vi "Write Resource.vi"(8 "error in (no error)":errorcluster, 10 "Resource":refnum<visa-resource-name>, 11 "Oscilloscope in":refnum<class "Oscilloscope.lvclass">) -> (0 "error out":errorcluster, 3 "Oscilloscope out":refnum<class "Oscilloscope.lvclass">)   [LabVIEW 2018, in "Oscilloscope.lvlib" / "Oscilloscope.lvclass"]
doc: "This acessor method writes resource ID setting."
uses:
  Oscilloscope.lvclass
  Oscilloscope.lvclass/Oscilloscope.ctl
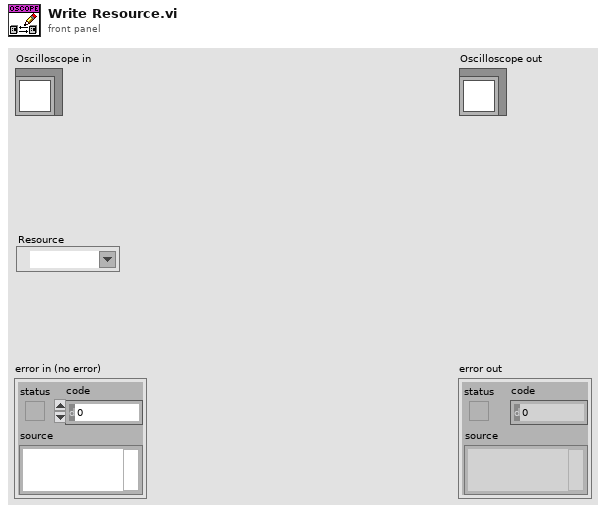
[diagram p1: front panel]
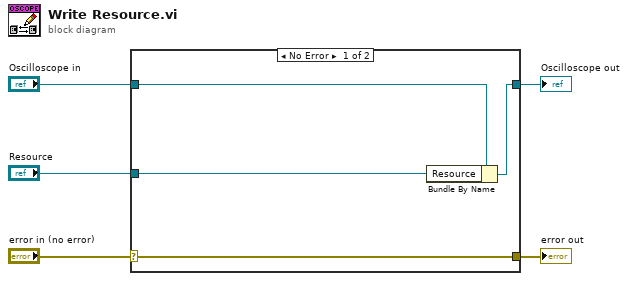
[diagram p0: block diagram]
diagram:
  n1 = case shown="No Error" "error in (no error)" {
    selector: "error in (no error)" -> [w9 w10]
    tunnel: [w9 w10] -> w4
    tunnel: [w7 w11] -> w2
    tunnel: "Oscilloscope in" -> [w8 w11]
    tunnel: "Resource" -> [w6 _]
    frame No Error {
      n2 = Bundle By Name(cluster=w8, "Resource"=w6) -> (w7:refnum<class "Oscilloscope.lvclass">)
    }
    frame Error {
    }
  }
  "error out" <- w4
  "Oscilloscope out" <- w2
